vi "WPI_SonarSRF04DigitalClose.vi"(8 "error in (no error)":errorcluster, 11 "UltrasonicDevRef":T1={"DevStatus"={"status"=FALSE, "code"=0, "source"=""}, "Ping Channel"=enum."Invalid", "Echo Channel"=enum."Invalid", "CntIndex"=enum."Invalid"}) -> (0 "error out":errorcluster)   [LabVIEW 2017]
doc: "Closes the reference to the ultrasonic sensor you specify. Use this VI to close each ultrasonic sensor reference that you open with the Open VI.\n\nThis software is licensed. Open the labview\\readme\\WPI Robotics Library Open Source License.txt file for more information."
uses:
  <vilib>/Rock Robotics/WPI/Ultrasonic/WPI_UltrasonicDeviceRef.ctl
  <vilib>/Rock Robotics/SystemInterfaces/DIO/FPGA_DIOChannel.ctl
  <vilib>/Rock Robotics/SystemInterfaces/Counter/FPGA_CounterCtrSystemIndex.ctl
  <instrlib>/Devantech SRF05/HAIOL/Devantech SRF05.lvclass
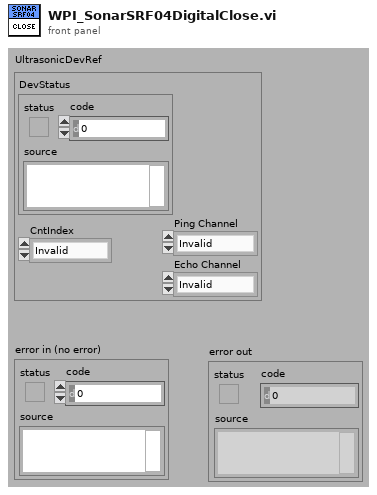
[diagram p1: front panel]
types:
  T1 = typedef "WPI_UltrasonicDeviceRef.ctl" = cluster{"DevStatus":errorcluster, "Ping Channel":T2, "Echo Channel":T2, "CntIndex":T3}
  T2 = typedef "FPGA_DIOChannel.ctl" = enum8{"DIO 0", "DIO 1", "DIO 2", "DIO 3", "DIO 4", "DIO 5", "DIO 6", "DIO 7", "DIO 8", "DIO 9", "DIO MXP 0", "DIO MXP 1", "DIO MXP 2", "DIO MXP 3", "DIO MXP 4", "DIO MXP 5", "DIO MXP 6", "DIO MXP 7", "DIO MXP 8", "DIO MXP 9", "DIO MXP 10", "DIO MXP 11", "DIO MXP 12", "DIO MXP 13", "DIO MXP 14", "DIO MXP 15", "SPI Port CS1", "SPI Port CS2", "SPI Port CS3", "SPI Port MISO", "SPI Port MOSI", "Invalid"}
  T3 = typedef "FPGA_CounterCtrSystemIndex.ctl" = enum8{"Ctr 0", "Ctr 1", "Ctr 2", "Ctr 3", "Ctr 4", "Ctr 5", "Ctr 6", "Ctr 7", "Invalid"}
  T4 = typedef "WPI_DigitalOutputDevRef.ctl" = cluster{"DIO Channel":T2, "DevStatus":errorcluster}
  T5 = typedef "WPI_CounterDevRef.ctl" = cluster{"DevStatus":errorcluster, "CntIndex":T3}
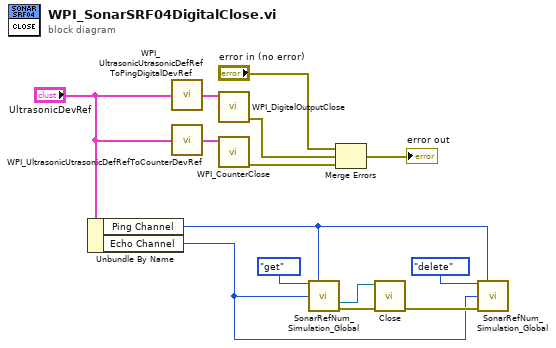
[diagram p0: block diagram]
diagram:
  n1 = Unbundle By Name("UltrasonicDevRef") -> ("Ping Channel"=w5:T2, "Echo Channel"=w1:T2)
  n2 = call <vilib>:"WPI_UltrasonicUtrasonicDefRefToPingDigitalDevRef.vi"("UltrasonicDevRef"="UltrasonicDevRef") -> ("DigitalOutputDevRef"=w13:T4)
  n3 = call <vilib>:"WPI_UltrasonicUtrasonicDefRefToCounterDevRef.vi"("UltrasonicDevRef"="UltrasonicDevRef") -> ("CounterDevRef in"=w14:T5)
  n4 = call <vilib>:"WPI_DigitalOutputClose.vi"("DigitalOutputDevRef"=w13) -> ("error out"=w11:errorcluster)  [unwired: 1 in, 9 out]
  n5 = call <vilib>:"WPI_CounterClose.vi"("CounterDevRef"=w14) -> ("error out"=w10:errorcluster)  [unwired: 2 in, 8 out]
  n6 = call <vilib>:"SonarRefNum_Simulation_Global.vi"("menu"=enum16{"set", "get", "delete"}."get", "Ping DIO Channel"=w5, "Echo DIO Channel"=w1) -> ("Devantech SRF05 Get"=w4:refnum<class "Devantech SRF05.lvclass">, "error out"=w3:errorcluster)  [unwired: 11 in]
  n7 = Merge Errors("error in (no error)", w11, w10) -> (→"error out":errorcluster)
  n8 = call-dynamic "Close.vi"("error in (no error)"=w3, "Devantech SRF05 in"=w4) -> ("error out"=w2:errorcluster)  [unwired: 9 in]
  n9 = call <vilib>:"SonarRefNum_Simulation_Global.vi"("menu"=enum16{"set", "get", "delete"}."delete", "Ping DIO Channel"=w5, "Echo DIO Channel"=w1, "error in (no error)"=w2) -> ()  [unwired: 10 in, 2 out]
